vi "Lab1FunGenOsc.vi"() -> ()   [LabVIEW 2015]
uses:
  <instrlib>/Siglent SDG 1000 5000 800 Series/Siglent SDG 1000 5000 800 Series.lvlib
  <instrlib>/Siglent SDS 1000 2000 Series/Siglent SDS 1000 2000 Series.lvlib
panel:
  in  "Parameter (P1: Amp, P2: Phase Shift)":u16(ring) items=["P1", "P2", "P3", "P4", "P5"]
  in  "Step Value":dbl=1000.0 min=1e-06 max=160000000.0 step=1.0 format="%#.6g"
  in  "Stop Value":dbl=1000.0 min=1e-06 max=160000000.0 step=1.0 format="%#.6g"
  in  "Start Value":dbl=1000.0 min=1e-06 max=160000000.0 step=1.0 format="%#.6g"
  out "Waveform Chart":dbl(graph)
  out "Amplitude/Phase Shift":dbl format="%#_3f"
  in  "Reset (True) 2":bool=TRUE
  in  "Reset (True)":bool=TRUE
  in  "error in (no error) 2":errorcluster
  in  "Oscilloscope":refnum<visa-resource-name>
  in  "error in (no error)":errorcluster
  in  "Function Generator":refnum<visa-resource-name>
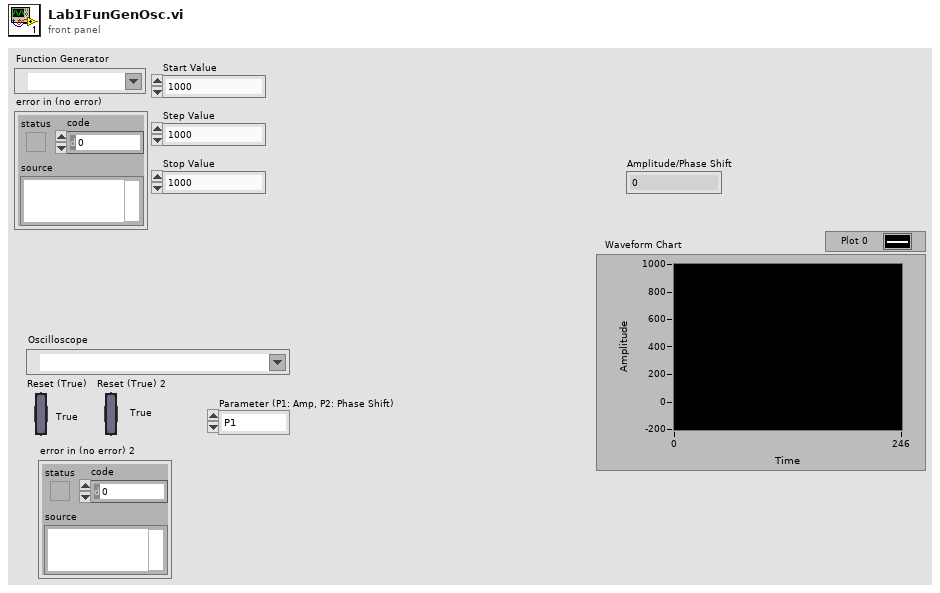
[diagram p1: front panel]
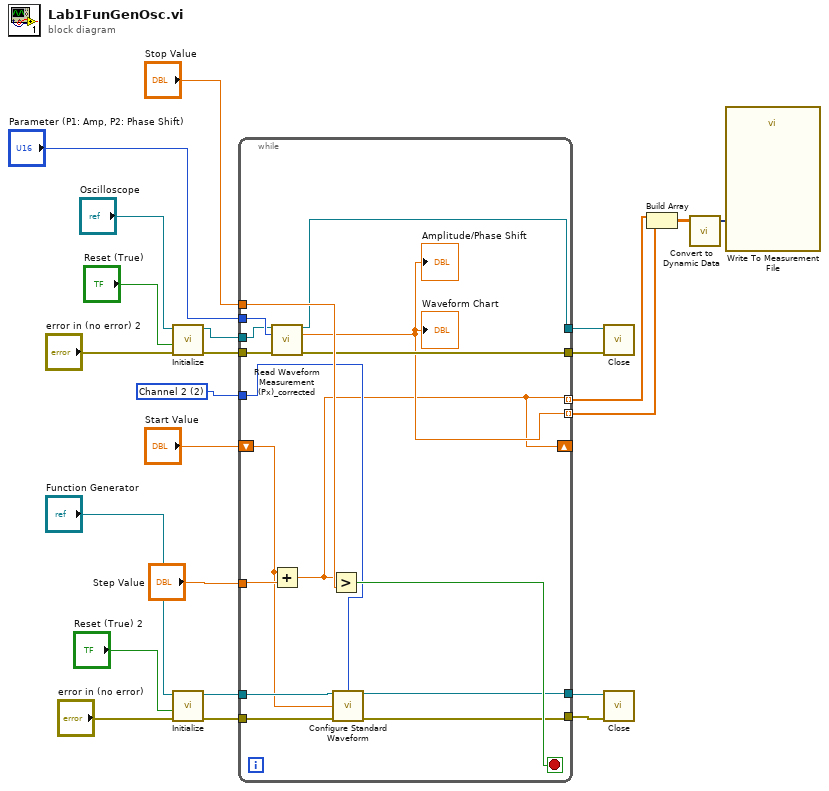
[diagram p0: block diagram]
diagram:
  w11 = 2 items=["Channel 1"=1, "Channel 2"=2] ("Channel (1:Channel 1)")
  n1 = call <instrlib>:"Initialize.vi"("error in (no error)"="error in (no error) 2", "Reset (True)"="Reset (True)", "VISA resource name"="Oscilloscope") -> ("error out"=w8:errorcluster, "VISA resource name out"=w6:refnum<visa-resource-name>)  [unwired: 7 in]
  n2 = call <instrlib>:"Initialize.vi"("error in (no error)"="error in (no error)", "Reset (True)"="Reset (True) 2", "VISA resource name"="Function Generator") -> ("error out"=w12:errorcluster, "VISA resource name out"=w15:refnum<visa-resource-name>)  [unwired: 7 in]
  n3 = while {
    tunnel: "Stop Value" -> [w39]
    tunnel: "Step Value" -> [w27]
    tunnel: w15 -> [w37]
    tunnel: [w36] -> w14
    tunnel: [w35] -> w13
    tunnel: w12 -> [w34]
    tunnel: w11 -> [w33]
    tunnel: [w30] -> w9
    tunnel: [w32] -> w10
    tunnel: w8 -> [w31]
    tunnel: [w24] -> w5 mode=indexing
    tunnel: "Parameter (P1: Amp, P2: Phase Shift)" -> [w29]
    tunnel: w6 -> [w28]
    tunnel: [w26] -> w4 mode=indexing
    shift-right: [w24] -> _
    shift-left: "Start Value" -> [w25]
    stop <- w38 stop-if-true
    n4 = call <instrlib>:"Read Waveform Measurement (Px)_corrected.vi"("VISA resource name"=w28, "Parameter (0: P1)"=w29, "error in (no error)"=w31) -> ("VISA resource name out"=w32:refnum<visa-resource-name>, "Value"=w26:dbl, "error out"=w30:errorcluster)  [unwired: 10 in]
    "Amplitude/Phase Shift" <- w26
    "Waveform Chart" <- w26
    n5 = Add(x=w25, y=w27) -> (x+y=w24:dbl)
    n6 = Greater?(x=w24, y=w39) -> (0:w38:bool)
    n7 = call <instrlib>:"Configure Standard Waveform.vi"("VISA resource name"=w37, "Channel (1:Channel 1)"=w33, "Frequency (1000 Hz)"=w25, "error in (no error)"=w34) -> ("VISA resource name out"=w36:refnum<visa-resource-name>, "error out"=w35:errorcluster)  [unwired: 10 in]
  }
  n8 = call <instrlib>:"Close.vi"("error in (no error)"=w9, "VISA resource name"=w10) -> ()  [unwired: 9 in, 1 out]
  n9 = call <instrlib>:"Close.vi"("error in (no error)"=w13, "VISA resource name"=w14) -> ()  [unwired: 9 in, 1 out]
  n10 = Build Array(w5, w4) -> (w3:dbl[][])
  n11 = call "Convert to Dynamic Data"("2D Array"=w3) -> ("Dynamic Data Type"=w2:dynamicdata)  [unwired: 3 in]
  n12 = call "Write To Measurement File"("Signals"=w2) -> ()  [unwired: 16 in, 3 out]
